vi "ClientConnectionInfo.vi"(8 "error in (no error)":errorcluster, 11 "AdsNET in":refnum<class "AdsNET.lvclass">) -> (0 "error out":errorcluster, 1 "ClientPort":i32, 2 "ClientNetID":string, 3 "AdsNET out":refnum<class "AdsNET.lvclass">)   [LabVIEW 2016, in "TCatAdsNet.lvlib" / "AdsNET.lvclass"]
doc: "Get ADS connection Client parameters."
uses:
  AdsNET.lvclass
  AdsNET.lvclass/AdsNET.ctl
  C:/Users/Maurizio/Projects/twincat-lv-ads-library/TCatAdsNet Library/TwinCAT.Ads.dll
  TwinCAT.Ads.dll
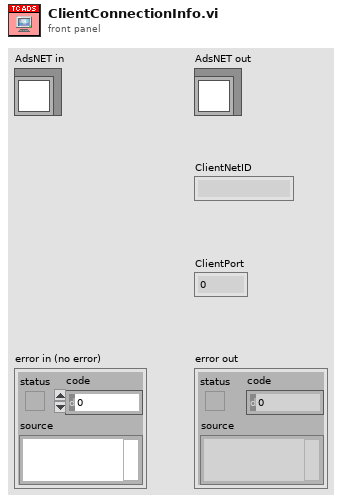
[diagram p1: front panel]
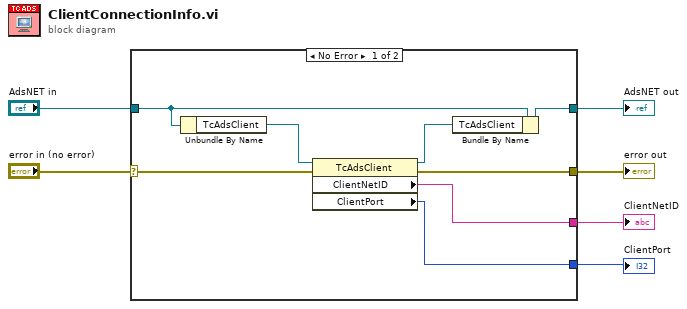
[diagram p0: block diagram]
diagram:
  n1 = case shown="No Error" "error in (no error)" {
    selector: "error in (no error)" -> [w12 w16]
    tunnel: [w11 w16] -> w5
    tunnel: [w10 w15] -> w3
    tunnel: "AdsNET in" -> [w14 w15]
    tunnel: [w8 _] -> w2
    tunnel: [w7 _] -> w1
    frame No Error {
      n2 = Unbundle By Name(w14) -> ("TcAdsClient"=w13:refnum<k24>)
      n3 = property class="TcAdsClient"(reference=w13, error in=w12) -> (reference out=w9:refnum<k24>, error out=w11:errorcluster, "ClientNetID"=w8:string, "ClientPort"=w7:i32)
      n4 = Bundle By Name(cluster=w14, "TcAdsClient"=w9) -> (w10:refnum<class "AdsNET.lvclass">)
    }
    frame Error {
    }
  }
  "error out" <- w5
  "AdsNET out" <- w3
  "ClientNetID" <- w2
  "ClientPort" <- w1
